vi "GetBonPeriod.vi"(8 "error in (no error)":errorcluster) -> (0 "error out":errorcluster, 3 "bonPeriodIn10ns0":u32)   [LabVIEW 2015, in "ESLSCDLL.lvlib"]
uses:
  ESLSCDLL.lvlib
  Globals.vi
panel:
  out "bonPeriodIn10ns1":u32
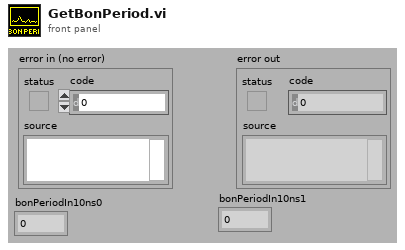
[diagram p1: front panel]
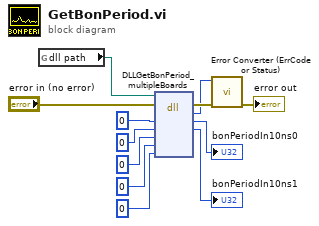
[diagram p0: block diagram]
diagram:
  n1 = global read "Globals.vi" "dll path"() -> (w1:path)
  n2 = dll-call lib="C:/ENTW/PCIE/LV64/board.vis/ESLSCDLL.dll" fn="DLLGetBonPeriod_multipleBoards" ("lwlscdll.dll:DLLWriteLongS0")(path in=w1, error in="error in (no error)", "bonPeriodIn10ns0"=u32 0 ("ADSC"), "bonPeriodIn10ns1"=u32 0 ("ADSC"), "bonPeriodIn10ns2"=u32 0 ("ADSC"), "bonPeriodIn10ns3"=u32 0 ("ADSC"), "bonPeriodIn10ns4"=u32 0 ("ADSC")) -> (error out=w10:errorcluster, "es_status_codes"=w9:i32, "bonPeriodIn10ns0"=→"bonPeriodIn10ns0":u32, "bonPeriodIn10ns1"=→"bonPeriodIn10ns1":u32)  [unwired: 4 in, 1 out]
  n3 = call "Error Converter (ErrCode or Status).vi"("error in (no error)"=w10, "error code"=w9) -> ("error out"=→"error out":errorcluster)  [unwired: 9 in]
